vi "Resample.vi"(8 "error in (no error)":errorcluster, 11 "Instrument.DAQ":refnum<class "Instrument.DAQ.lvclass">) -> (0 "error out":errorcluster, 3 "Instrument.DAQ out":refnum<class "Instrument.DAQ.lvclass">)   [LabVIEW 2019, in "Instrument.Lockin.lvlib" / "Instrument.DAQ.lvclass"]
uses:
  Instrument.DAQ.lvclass
  Instrument.DAQ.lvclass/Instrument.DAQ.ctl
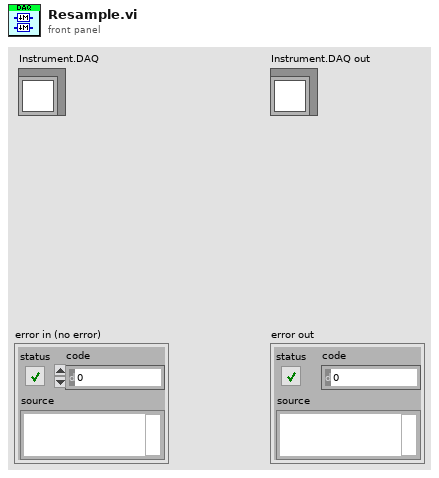
[diagram p1: front panel]
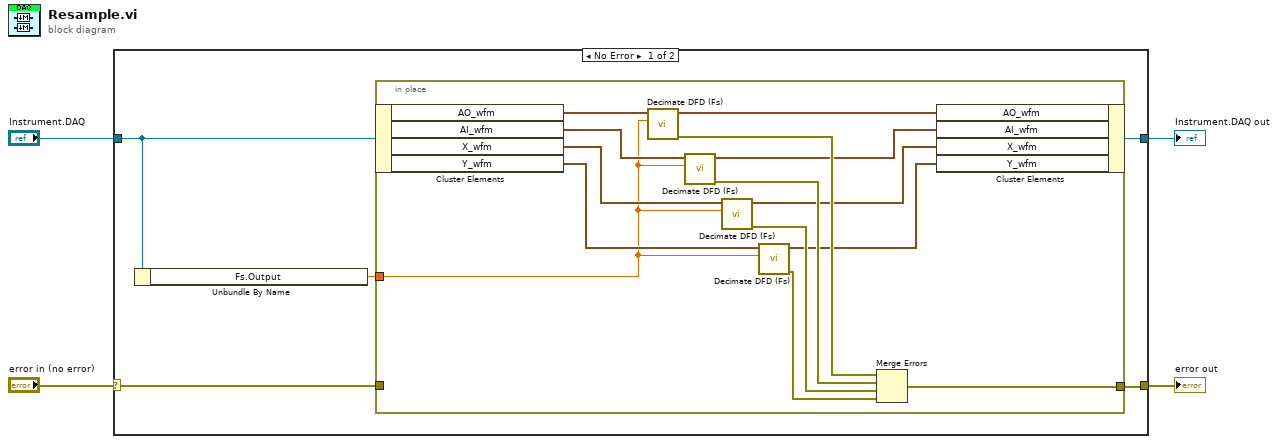
[diagram p0: block diagram]
diagram:
  n1 = case shown="No Error" "error in (no error)" {
    selector: "error in (no error)" -> [w9 w25]
    tunnel: [w7 w25] -> w3
    tunnel: "Instrument.DAQ" -> [w8 w24]
    tunnel: [w6 w24] -> w1
    frame No Error {
      n2 = Unbundle By Name(w8) -> ("Fs.Output"=w5:dbl)
      n3 = in-place {
        in-place-border: w9 -> [_]
        in-place-border: [w23] -> w7
        in-place-border: w5 -> [w10]
        n4 = in-place-cluster #1(w8) -> ("AO_wfm"=w18:waveform(dbl)[], "AI_wfm"=w17:waveform(dbl)[], "X_wfm"=w16:waveform(dbl)[], "Y_wfm"=w15:waveform(dbl)[])
        n5 = call "Decimate DFD (Fs).vi"("output fs[Hz]"=w10, "Waveforms in"=w18) -> ("error out"=w22:errorcluster, "waveforms out"=w14:waveform(dbl)[])  [unwired: 8 in]
        n6 = call "Decimate DFD (Fs).vi"("output fs[Hz]"=w10, "Waveforms in"=w17) -> ("error out"=w21:errorcluster, "waveforms out"=w13:waveform(dbl)[])  [unwired: 8 in]
        n7 = call "Decimate DFD (Fs).vi"("output fs[Hz]"=w10, "Waveforms in"=w16) -> ("error out"=w20:errorcluster, "waveforms out"=w12:waveform(dbl)[])  [unwired: 8 in]
        n8 = call "Decimate DFD (Fs).vi"("output fs[Hz]"=w10, "Waveforms in"=w15) -> ("error out"=w19:errorcluster, "waveforms out"=w11:waveform(dbl)[])  [unwired: 8 in]
        n9 = Merge Errors(w22, w21, w20, w19) -> (w23:errorcluster)
        n10 = in-place-cluster #1("AO_wfm"=w14, "AI_wfm"=w13, "X_wfm"=w12, "Y_wfm"=w11) -> (w6:refnum<class "Instrument.DAQ.lvclass">)
      }
    }
    frame Error {
    }
  }
  "error out" <- w3
  "Instrument.DAQ out" <- w1
